vi "Arm Tellescope.vi"(6 "C Button":bool, 7 "B Button":bool, 8 "A Button":bool, 9 "Arm Tellescope Manuel Control":dbl format="%#_13g") -> ()   [LabVIEW 2020]
uses:
  <vilib>/Rock Robotics/WPI/ThirdParty/Phoenix-LabVIEW/Motor Controller/Controls/CTRE_Phoenix_MotorControl_ControlMode.ctl
panel:
  in  "Arm Tellescope Set Value":dbl
  out "Arrived At Setpoint":bool
  in  "Arm Tellescope Value":dbl
  out "Where is Arm Tellescope":dbl(graph)
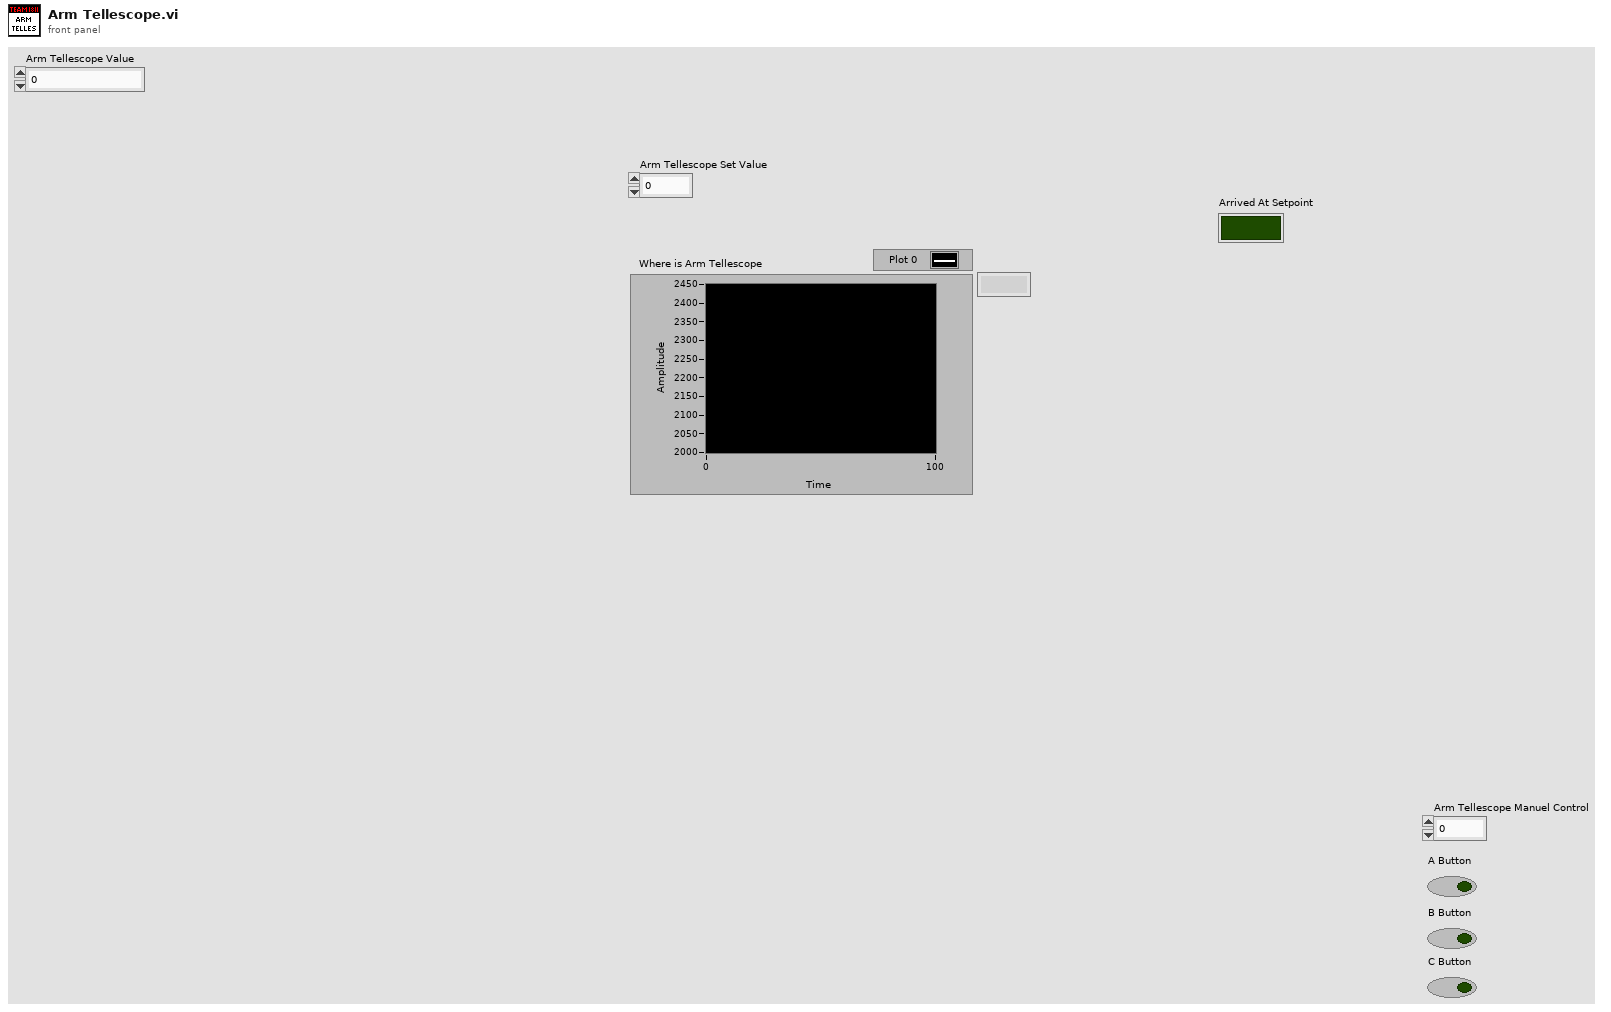
[diagram p1: front panel]
types:
  T1 = typedef "CTRE_Phoenix_MotorControl_ControlMode.ctl" = u16
  T2 = typedef "WPI_MotorControlDeviceRef.ctl" = cluster{"DeviceStatus":errorcluster, "Type":T3, "PWM":cluster{"PWM Channel":T4, "DeadBand":T5}, "CAN":cluster{"Device Number":u8, "SetOutput VI Ref":variant, "GetOutput VI Ref":variant, "Enable VI Ref":variant, "Disable VI Ref":variant, "Data":variant}, "Invert":bool, "DIO PWM":cluster{"PWM \"Enable\" Channel":T4, "DIOChannel":T6, "PWM Rate":dbl}}
  T3 = typedef "WPI_MotorControlType.ctl" = enum16{"PWM", "CAN", "DIO PWM"}
  T4 = typedef "FPGA_DIOPWMChannel.ctl" = enum8{"PWM 0", "PWM 1", "PWM 2", "PWM 3", "PWM 4", "PWM 5", "PWM 6", "PWM 7", "PWM 8", "PWM 9", "PWM MXP 0", "PWM MXP 1", "PWM MXP 2", "PWM MXP 3", "PWM MXP 4", "PWM MXP 5", "PWM MXP 6", "PWM MXP 7", "PWM MXP 8", "PWM MXP 9", "Invalid"}
  T5 = typedef "WPI_PWMDeadband.ctl" = cluster{"Name":string, "maxPositivePwm":i32, "minPositivePwm":i32, "centerPwm":i32, "maxNegativePwm":i32, "minNegativePwm":i32, "angularRange":u16}
  T6 = typedef "FPGA_DIOChannel.ctl" = enum8{"DIO 0", "DIO 1", "DIO 2", "DIO 3", "DIO 4", "DIO 5", "DIO 6", "DIO 7", "DIO 8", "DIO 9", "DIO MXP 0", "DIO MXP 1", "DIO MXP 2", "DIO MXP 3", "DIO MXP 4", "DIO MXP 5", "DIO MXP 6", "DIO MXP 7", "DIO MXP 8", "DIO MXP 9", "DIO MXP 10", "DIO MXP 11", "DIO MXP 12", "DIO MXP 13", "DIO MXP 14", "DIO MXP 15", "SPI Port CS1", "SPI Port CS2", "SPI Port CS3", "SPI Port MISO", "SPI Port MOSI", "Invalid"}
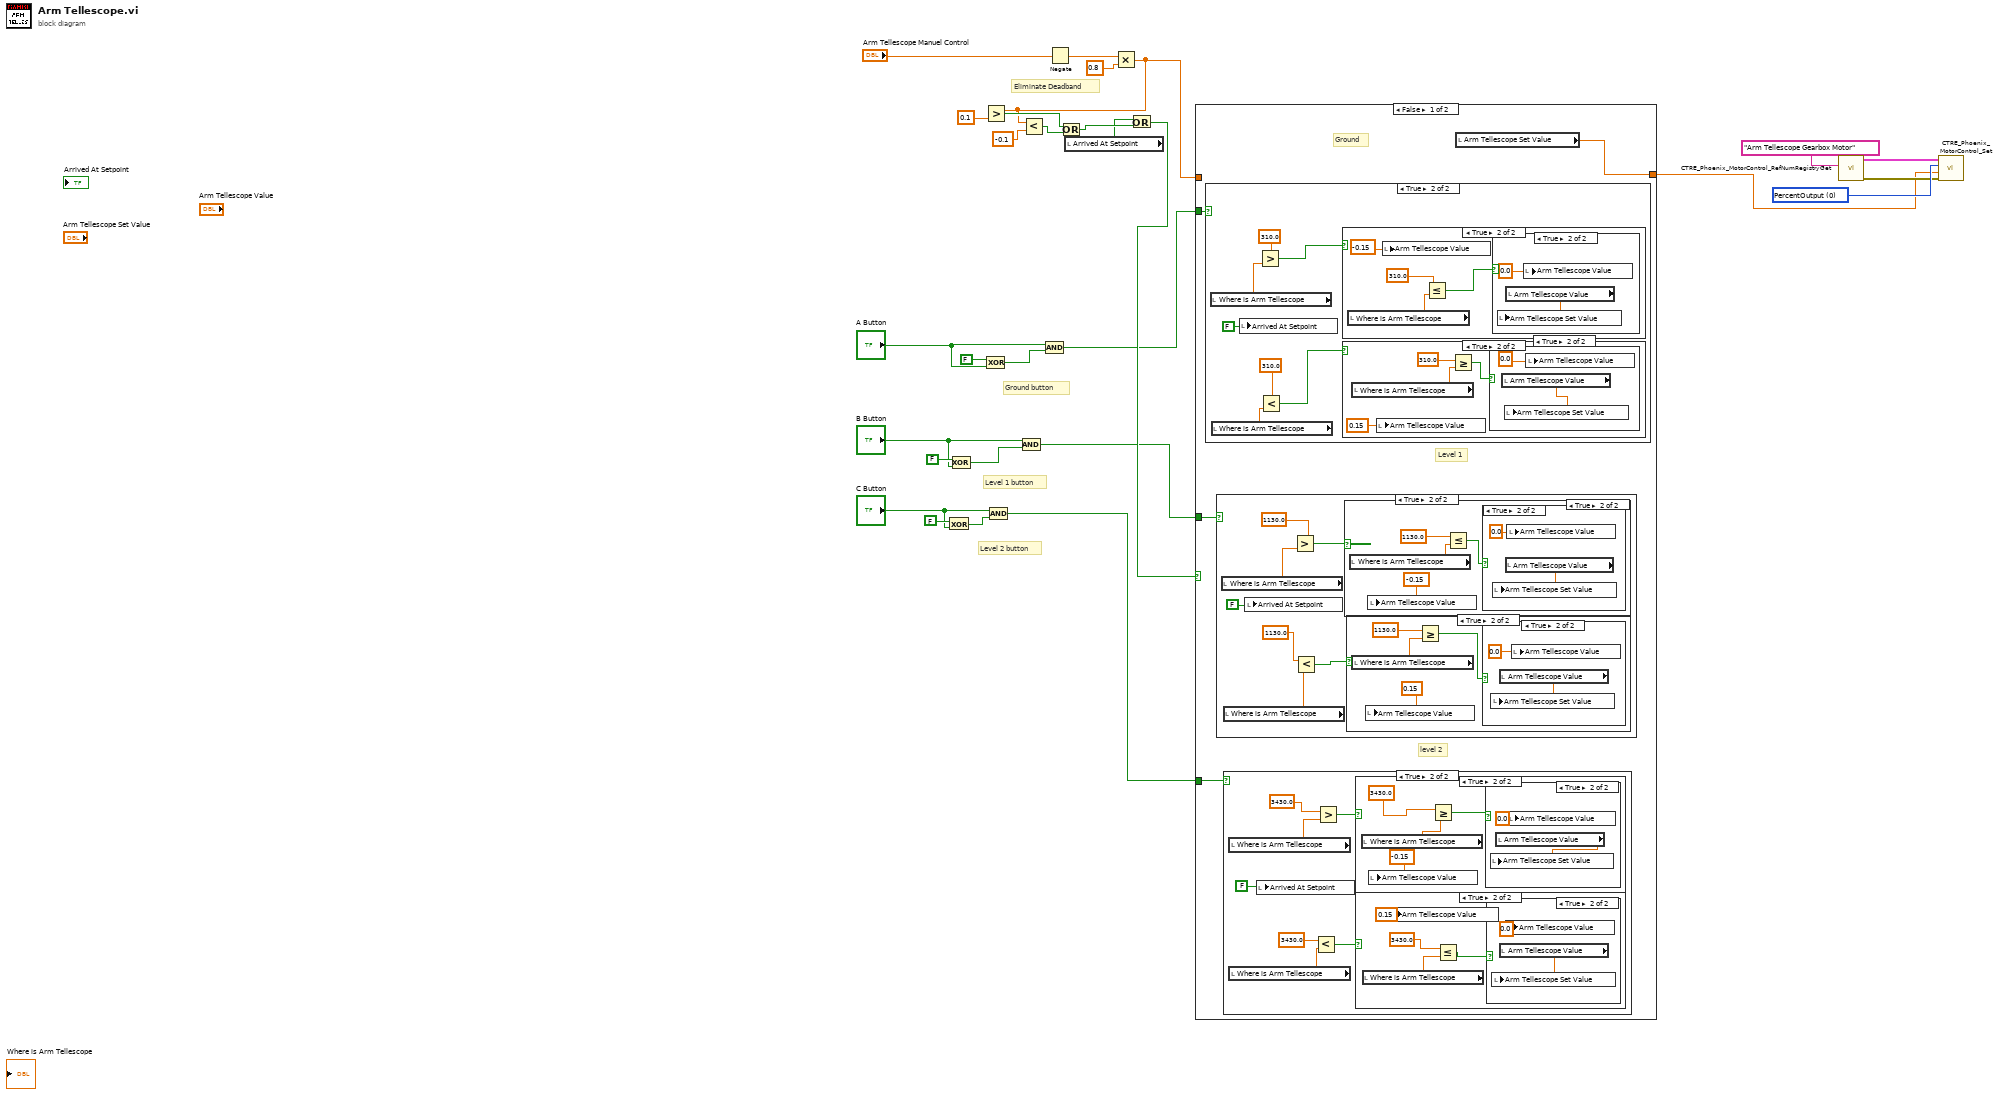
[diagram p0: block diagram]
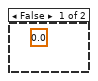
[diagram p12: hidden frame]
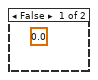
[diagram p15: hidden frame]
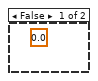
[diagram p16: hidden frame]
diagram:
  w6 = T1 0 items=["PercentOutput"=0, "Position"=1, "Velocity"=2, "Current"=3, "Follower"=5, "MotionProfile"=6, "MotionMagic"=7, "MotionProfileArc"=10, "Disabled"=15] ("Control Mode")
  # "Level 2 button"
  # "Level 1 button"
  # "Ground button"
  # "Eliminate Deadband"
  n1 = Exclusive Or(1:"C Button", 2:FALSE ("x")) -> (0:w28:bool)
  n2 = Exclusive Or(1:"B Button", 2:FALSE ("x")) -> (0:w27:bool)
  n3 = Exclusive Or(1:"A Button", 2:FALSE ("x")) -> (0:w12:bool)
  n4 = And(x="C Button", y=w28) -> (x .and. y?=w11:bool)
  n5 = And(x="B Button", y=w27) -> (x .and. y?=w14:bool)
  n6 = And(x="A Button", y=w12) -> (x .and. y?=w13:bool)
  n7 = Negate(x="Arm Tellescope Manuel Control") -> (-x=w26:dbl)
  n8 = local read "Arrived At Setpoint"() -> (w19:bool)
  n9 = Multiply(x=w26, y=0.8) -> (x*y=w1:dbl)
  n10 = Greater?(x=w1, y=0.1) -> (0:w22:bool)
  n11 = Less?(x=w1, y=-0.1) -> (x < y?=w23:bool)
  n12 = Or(x=w22, y=w23) -> (x .or. y?=w21:bool)
  n13 = Or(x=w19, y=w21) -> (x .or. y?=w15:bool)
  n14 = case shown="False" w15 {
    tunnel: w1 -> [_ w90]
    tunnel: w13 -> [w32 _]
    tunnel: w14 -> [w31 _]
    tunnel: w11 -> [w30 _]
    tunnel: [w29 w90] -> w2
    frame False {
      # "Level 1"
      # "Ground"
      # "level 2"
      n15 = case shown="True" w32 {
        frame False {
          (unwired) 0.0
        }
        frame True {
          n16 = local read "Where is Arm Tellescope"() -> (w74:dbl)
          n17 = local read "Where is Arm Tellescope"() -> (w77:dbl)
          n18 = local write "Arrived At Setpoint"(FALSE) -> ()
          n19 = Greater?(x=310.0, y=w74) -> (0:w73:bool)
          n20 = Less?(x=310.0, y=w77) -> (x < y?=w72:bool)
          n21 = case shown="True" w73 {
            frame False {
              (unwired) 0.0
            }
            frame True {
              n22 = local read "Where is Arm Tellescope"() -> (w86:dbl)
              n23 = local write "Arm Tellescope Value"(-0.15 ("Position Telloscoping arm")) -> ()
              n24 = Less Or Equal?(x=310.0, y=w86) -> (x <= y?=w84:bool)
              n25 = case shown="True" w84 {
                frame False {
                  (unwired) 0.0
                }
                frame True {
                  n26 = local read "Arm Tellescope Value"() -> (w88:dbl)
                  n27 = local write "Arm Tellescope Set Value"(w88) -> ()
                  n28 = local write "Arm Tellescope Value"(0.0 ("Arm Tellescope")) -> ()
                }
              }
            }
          }
          n29 = case shown="True" w72 {
            frame False {
            }
            frame True {
              n30 = local read "Where is Arm Tellescope"() -> (w79:dbl)
              n31 = local write "Arm Tellescope Value"(0.15 ("Arm Movement")) -> ()
              n32 = Greater Or Equal?(x=310.0, y=w79) -> (x >= y?=w78:bool)
              n33 = case shown="True" w78 {
                frame False {
                }
                frame True {
                  n34 = local read "Arm Tellescope Value"() -> (w82:dbl)
                  n35 = local write "Arm Tellescope Set Value"(w82) -> ()
                  n36 = local write "Arm Tellescope Value"(0.0 ("Arm Tellescope")) -> ()
                }
              }
            }
          }
        }
      }
      n37 = case shown="True" w31 {
        frame False {
        }
        frame True {
          n38 = local read "Where is Arm Tellescope"() -> (w54:dbl)
          n39 = local read "Where is Arm Tellescope"() -> (w53:dbl)
          n40 = local write "Arrived At Setpoint"(FALSE) -> ()
          n41 = Greater?(x=1130.0, y=w54) -> (0:w55:bool)
          n42 = Less?(x=1130.0, y=w53) -> (x < y?=w56:bool)
          n43 = case shown="True" w55 {
            frame False {
            }
            frame True {
              n44 = local read "Where is Arm Tellescope"() -> (w61:dbl)
              n45 = local write "Arm Tellescope Value"(-0.15) -> ()
              n46 = Less Or Equal?(x=1130.0, y=w61) -> (x <= y?=w59:bool)
              n47 = case shown="True" w59 {
                frame False {
                }
                frame True {
                  n48 = local read "Arm Tellescope Value"() -> (w63:dbl)
                  n49 = local write "Arm Tellescope Set Value"(w63) -> ()
                  n50 = local write "Arm Tellescope Value"(0.0) -> ()
                }
              }
            }
          }
          n51 = case shown="True" w56 {
            frame False {
            }
            frame True {
              n52 = local read "Where is Arm Tellescope"() -> (w67:dbl)
              n53 = local write "Arm Tellescope Value"(0.15 ("Arm Motor Position")) -> ()
              n54 = Greater Or Equal?(x=1130.0, y=w67) -> (x >= y?=w65:bool)
              n55 = case shown="True" w65 {
                frame False {
                }
                frame True {
                  n56 = local read "Arm Tellescope Value"() -> (w69:dbl)
                  n57 = local write "Arm Tellescope Set Value"(w69) -> ()
                  n58 = local write "Arm Tellescope Value"(0.0 ("Position Telloscoping arm")) -> ()
                }
              }
            }
          }
        }
      }
      n59 = case shown="True" w30 {
        frame False {
        }
        frame True {
          n60 = local read "Where is Arm Tellescope"() -> (w34:dbl)
          n61 = local read "Where is Arm Tellescope"() -> (w36:dbl)
          n62 = local write "Arrived At Setpoint"(FALSE) -> ()
          n63 = Less?(x=3430.0, y=w36) -> (x < y?=w38:bool)
          n64 = Greater?(x=3430.0, y=w34) -> (0:w35:bool)
          n65 = case shown="True" w35 {
            frame False {
            }
            frame True {
              n66 = local read "Where is Arm Tellescope"() -> (w43:dbl)
              n67 = local write "Arm Tellescope Value"(-0.15) -> ()
              n68 = Greater Or Equal?(x=3430.0, y=w43) -> (x >= y?=w40:bool)
              n69 = case shown="True" w40 {
                frame False {
                }
                frame True {
                  n70 = local read "Arm Tellescope Value"() -> (w44:dbl)
                  n71 = local write "Arm Tellescope Set Value"(w44) -> ()
                  n72 = local write "Arm Tellescope Value"(0.0) -> ()
                }
              }
            }
          }
          n73 = case shown="True" w38 {
            frame False {
            }
            frame True {
              n74 = local read "Where is Arm Tellescope"() -> (w48:dbl)
              n75 = local write "Arm Tellescope Value"(0.15 ("Arm Motor Position")) -> ()
              n76 = Less Or Equal?(x=3430.0, y=w48) -> (x <= y?=w46:bool)
              n77 = case shown="True" w46 {
                frame False {
                }
                frame True {
                  n78 = local read "Arm Tellescope Value"() -> (w50:dbl)
                  n79 = local write "Arm Tellescope Set Value"(w50) -> ()
                  n80 = local write "Arm Tellescope Value"(0.0 ("Position Telloscoping arm")) -> ()
                }
              }
            }
          }
        }
      }
      n81 = local read "Arm Tellescope Set Value"() -> (w29:dbl)
    }
    frame True {
      # "Give Control To Driver Joystick"
    }
  }
  n82 = call <vilib>:"CTRE_Phoenix_MotorControl_RefNumRegistryGet.vi"("refnum name"="Arm Tellescope Gearbox Motor") -> ("error out"=w4:errorcluster, "PhoenixMotorControlDevRef"=w5:T2)  [unwired: 9 in]
  n83 = call <vilib>:"CTRE_Phoenix_MotorControl_Set.vi"("error in (no error)"=w4, "Output"=w2, "Control Mode"=w6, "PhoenixMotorControlDevRef"=w5) -> ()  [unwired: 6 in, 2 out]
